vi "添加MN号.vi"(8 "error in (no error)":errorcluster caption="错误输入（无错误）", 11 "簇":cluster{"MN":string, "PW":string}={"MN"="平台数据发送系统", "PW"="平台数据发送系统"}) -> (0 "error out":errorcluster caption="错误输出", 3 "添加成功标记":bool)   [LabVIEW 2016, in "数据传输系统-03.lvlib"]
uses:
  <vilib>/registry/registry.llb/Registry RtKey.ctl
  <vilib>/registry/registry.llb/Write Registry Value Simple STR.vi
panel:
  out "值":string[](array[string])
  out "名称":string[](array[string])
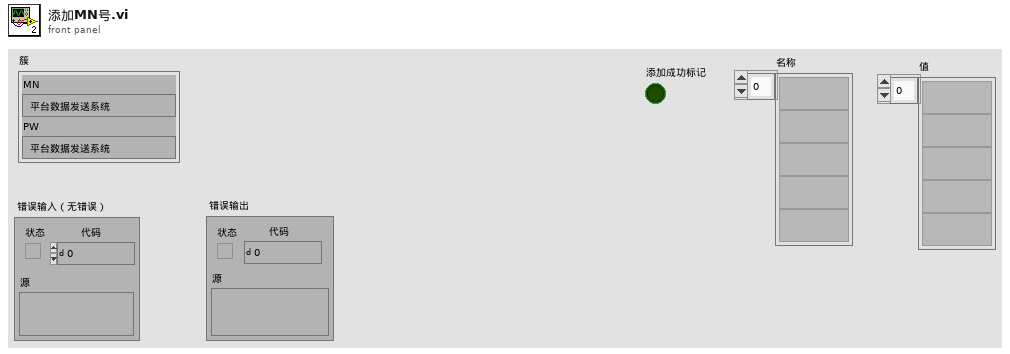
[diagram p1: front panel]
types:
  T1 = typedef "Registry RtKey.ctl" = enum32{"HKEY_CLASSES_ROOT", "HKEY_CURRENT_USER", "HKEY_LOCAL_MACHINE", "HKEY_USERS", "HKEY_PERFORMANCE_DATA", "HKEY_CURRENT_CONFIG", "HKEY_DYN_DATA"}
  T2 = typedef "Registry refnum.ctl" = refnum<k1>
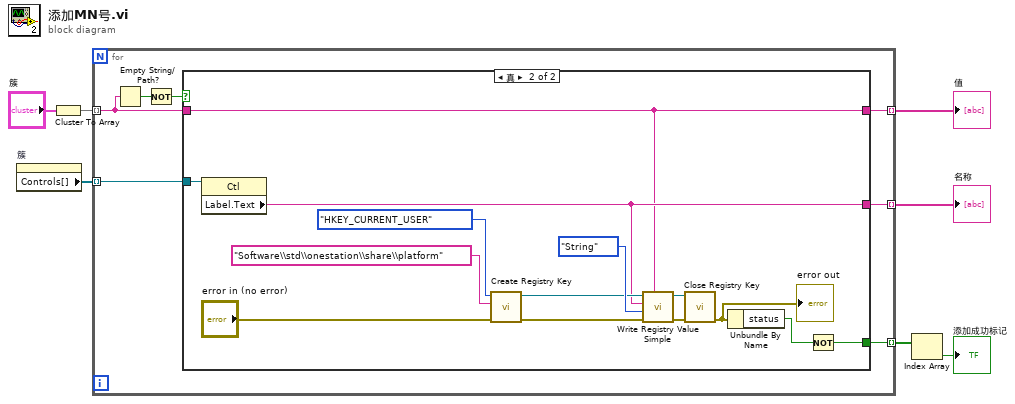
[diagram p0: block diagram]
diagram:
  n1 = property on="簇" class="Clust (严格)"() -> ("Controls[]"=w5:refnum<vi>[])  [unwired: 2 in, 2 out]
  n2 = Cluster To Array(cluster="簇") -> (array=w6:string[])
  n3 = for {
    tunnel: w6 -> [w12] mode=indexing
    tunnel: w5 -> [w11] mode=indexing
    tunnel: [w10] -> w4 mode=indexing
    tunnel: [w9] -> w3 mode=indexing
    tunnel: [w8] -> w2 mode=indexing
    n4 = Empty String/Path?(string/path=w12) -> (empty?=w14:bool)
    n5 = Not(x=w14) -> (.not. x?=w13:bool)
    n6 = case shown="真" w13 {
      tunnel: w12 -> [_ w15]
      tunnel: [_ w23] -> w8
      tunnel: w11 -> [_ w17]
      tunnel: [_ w16] -> w10
      tunnel: [_ w15] -> w9
      frame False {
      }
      frame True {
        n7 = property class="Ctl"(reference=w17) -> ("Label.Text"=w16:string)  [unwired: 1 in, 2 out]
        n8 = call <vilib>:"Create Registry Key.vi"("error in (no error)"="error in (no error)", "subkey"="Software\\std\\onestation\\share\\platform", "root key (HKEY_LOCAL_MACHINE)"=Registry_RtKey."HKEY_CURRENT_USER") -> ("error out"=w19:errorcluster, "refnum out"=w20:T2)  [unwired: 6 in, 1 out]
        n9 = call-poly <vilib>:"Write Registry Value Simple.vi"("String/Binary data"=w15, "error in (no error)"=w19, "simple data type"=enum16{"String", "Binary", "DWORD"}."String", "value"=w16, "refnum"=w20) -> ("error out"=w28:errorcluster, "refnum out"=w27:T2)  [unwired: 3 in]
        n10 = call <vilib>:"Close Registry Key.vi"("error in (no error)"=w28, "refnum"=w27) -> ("error out"=w25:errorcluster)  [unwired: 5 in]
        "error out" <- w25
        n11 = Unbundle By Name(w25) -> ("status"=w24:bool)
        n12 = Not(x=w24) -> (.not. x?=w23:bool)
      }
    }
  }
  "名称" <- w4
  "值" <- w3
  n13 = Index Array(array=w2) -> (element=→"添加成功标记":bool)  [unwired: 1 in]
